vi "LabviewCamCode.vi"() -> ()   [LabVIEW 2026]
doc: "The Acquire Most Recent Image (Express VI) example acquires images continuously and displays the images in an image control using the Vision Acquisition Express VI. The Express VI makes configuring acquisitions simple and allows you to change the selected camera, or add new attributes or settings to update without writing any code. This Express VI is appropriate for getting started and learning how to acquire images from a camera and display the images in LabVIEW."
uses:
  Instance           1 22Saved   Grab (Express) .vi
panel:
  out "Frame Rate":dbl
  out "Buffer Number":u32
  out "Image":T1(plugin-control)
  in  "Stop":bool
  # "Overview: Demonstrates how to acquire images continuously using an Express VI.\nRequirements: Vision Acquisition Software\nInstructions: Run the VI"
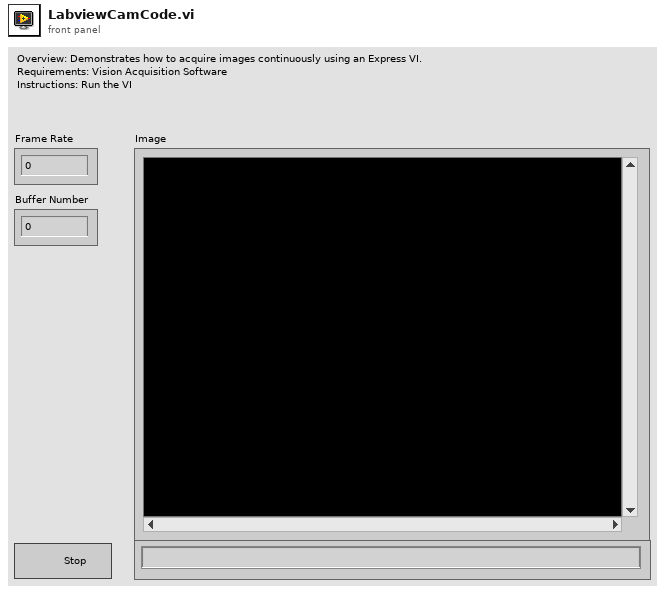
[diagram p1: front panel]
types:
  T1 = typedef "IMAQ Image.ctl" = refnum<image>
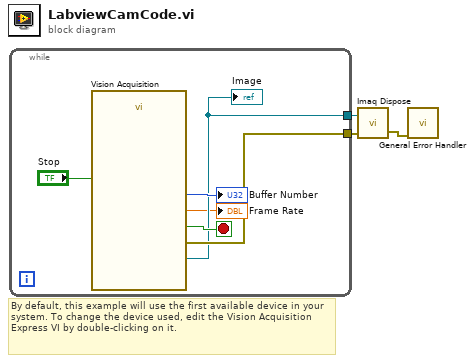
[diagram p0: block diagram]
diagram:
  # "By default, this example will use the first available device in your system. To change the device used, edit the Vision Acquisition Express VI by double-clicking on it."
  n1 = while {
    tunnel: [w6] -> w3
    tunnel: [w5] -> w1
    stop <- w9 stop-if-true
    n2 = call "Vision Acquisition"("Stop (F)"="Stop") -> ("Image Out"=w5:T1, "Image Number"=→"Buffer Number":u32, "Frame Rate"=→"Frame Rate":dbl, "Stopped"=w9:bool, "error out"=w6:errorcluster)  [unwired: 1 in, 21 out]
    "Image" <- w5
  }
  n3 = call "Imaq Dispose"("Image"=w1, "error in (no error)"=w3) -> ("error out"=w2:errorcluster)  [unwired: 4 in]
  n4 = call <vilib>:"General Error Handler.vi"("error in (no error)"=w2) -> ()  [unwired: 2 in, 13 out]
